vi "CSV File Logging Example.vi"() -> ()   [LabVIEW 2014]
panel:
  in  "Cooling Parameters":cluster{"dt":dbl, "T0":dbl, "Tf":dbl, "k":dbl}={"dt"=0.1, "T0"=10.0, "Tf"=1.0, "k"=0.1}
  in  "stop":bool
  out "Time Stamp":timestamp
  in  "File Path":path
  in  "Comment":string="Testing file writing"
  out "Waveform Chart":T1(graph)
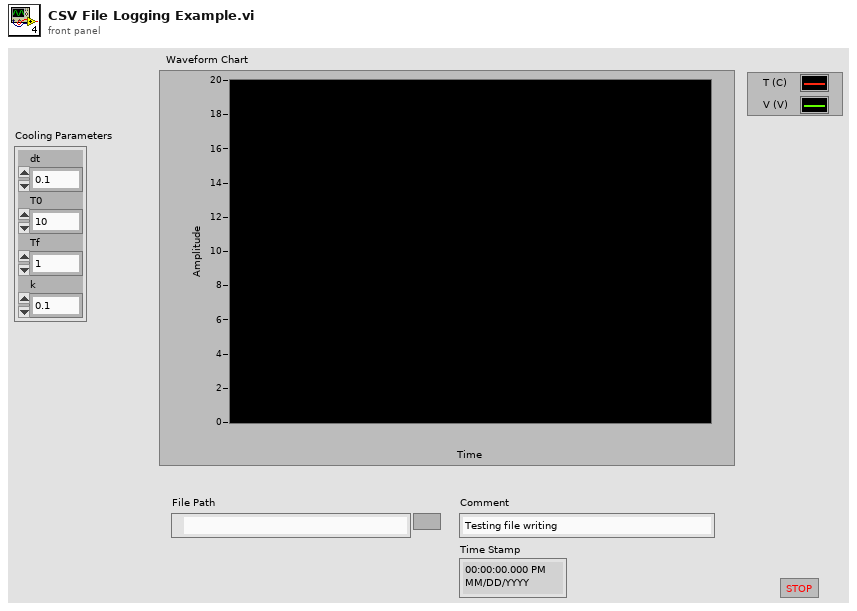
[diagram p1: front panel]
types:
  T1 = cluster{"Temperature (C)":dbl, "Voltage (V)":dbl}
  T2 = cluster{"Time (s)":dbl, "Temperature (C)":dbl, "Voltage (V)":dbl}
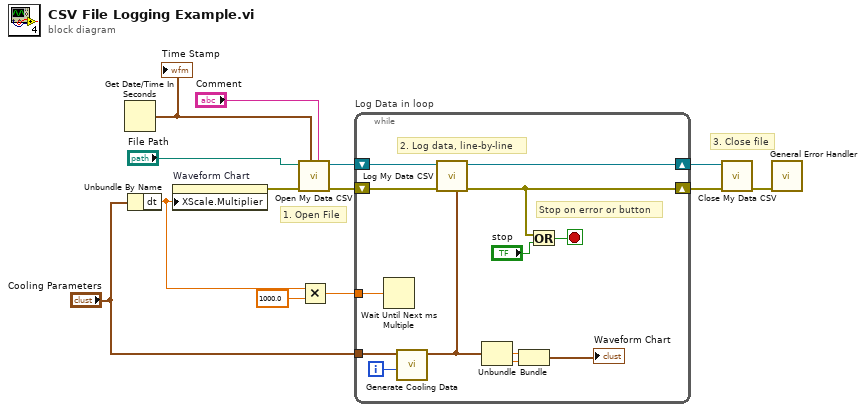
[diagram p0: block diagram]
diagram:
  # "3. Close file"
  # "1. Open File"
  n1 = Get Date/Time In Seconds() -> (seconds since 1Jan1904=w11:timestamp)
  "Time Stamp" <- w11
  n2 = Unbundle By Name("Cooling Parameters") -> ("dt"=w3:dbl)
  n3 = property on="Waveform Chart" class="WFChart (strict)"("XScale.Multiplier"=w3) -> (error out=w12:errorcluster)  [unwired: 2 in, 1 out]
  n4 = call "Open My Data CSV.vi"("Comment"="Comment", "Time Stamp"=w11, "error in"=w12, "file path"="File Path") -> ("error out"=w8:errorcluster, "refnum out"=w7:refnum<file>)  [unwired: 6 in]
  n5 = Multiply(x=w3, y=1000.0) -> (x*y=w1:dbl)
  n6 = while "Log Data in loop" {
    tunnel: "Cooling Parameters" -> [w25]
    shift-right: [w16] -> w6
    shift-left: w8 -> [w18]
    shift-right: [w15] -> w5
    shift-left: w7 -> [w19]
    tunnel: w1 -> [w14]
    i -> [w26]
    stop <- w20 stop-if-true
    # "2. Log data, line-by-line"
    # "Stop on error or button"
    n7 = Wait Until Next ms Multiple(millisecond multiple=w14) -> ()  [unwired: 1 out]
    n8 = call "Generate Cooling Data.vi"("i"=w26, "Cooling Parameters"=w25) -> ("Data"=w17:T2)  [unwired: 9 in]
    n9 = call "Log My Data CSV.vi"("Data element"=w17, "error in"=w18, "file refnum"=w19) -> ("error out"=w16:errorcluster, "file refnum out"=w15:refnum<file>)  [unwired: 7 in]
    n10 = Unbundle(w17) -> ("Temperature (C)"=w24:dbl, "Voltage (V)"=w23:dbl)  [unwired: 1 out]
    n11 = Bundle("Temperature (C)"=w24, "Voltage (V)"=w23) -> (→"Waveform Chart":T1)  [unwired: 1 in]
    n12 = Or(x=w16, y="stop") -> (x .or. y?=w20:bool)
  }
  n13 = call "Close My Data CSV.vi"("error in"=w6, "file refnum"=w5) -> ("error out"=w4:errorcluster)  [unwired: 9 in]
  n14 = call <vilib>:"General Error Handler.vi"("error in (no error)"=w4) -> ()  [unwired: 10 in, 5 out]
